vi "UTILITY Find Sigma Limit.vi"(8 "Error In":errorcluster, 11 "Filtered Power Data (W)":dbl[](array[numeric])) -> (0 "Error Out":errorcluster, 1 "Lower 3 Sig Limit":dbl, 2 "Upper 3 Sig Limit":dbl, 3 "Average Compressor Power (Watts)":dbl format="%0.2f")   [LabVIEW 2016]
uses:
  <vilib>/Analysis/baseanly.llb/Mean (DBL).vi
  <vilib>/gmath/NI_Gmath.lvlib
  <vilib>/Analysis/NI_AALBase.lvlib
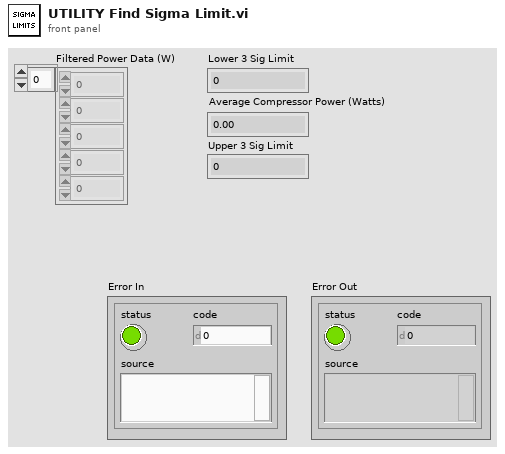
[diagram p1: front panel]
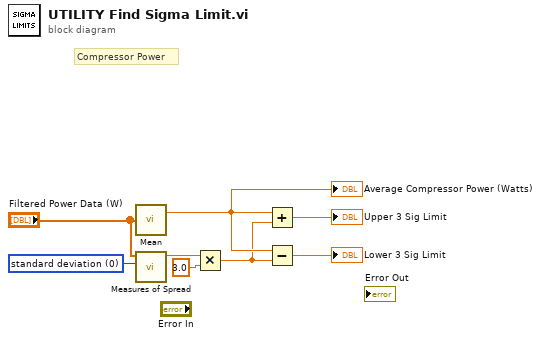
[diagram p0: block diagram]
diagram:
  w5 = 0 items=["standard deviation", "range", "mean absolute deviation", "interquartile range"] ("type")
  # "Compressor Power"
  n1 = call-poly <vilib>:"Mean.vi"("X"="Filtered Power Data (W)") -> ("mean"=w2:dbl)  [unwired: 1 out]
  "Average Compressor Power (Watts)" <- w2
  n2 = call <vilib>:"Measures of Spread.vi"("type"=w5, "x array"="Filtered Power Data (W)") -> ("spread value"=w4:dbl)  [unwired: 8 in, 1 out]
  n3 = Multiply(x=w4, y=3.0) -> (x*y=w1:dbl)
  n4 = Add(x=w2, y=w1) -> (x+y=→"Upper 3 Sig Limit":dbl)
  n5 = Subtract(x=w2, y=w1) -> (x-y=→"Lower 3 Sig Limit":dbl)
